vi "OperateOnDigitalOutput.vi"(2 "error in (no error)":errorcluster, 3 "Image Settings":T1={"Start Position (µm)"={"x"=0.0, "y"=0.0, "z"=0.0}, "End Position (µm)"={"x"=10.0, "y"=10.0, "z"=0.0}, "Image Resolution (nm/pixel)"={"x"=50.0, "y"=50.0, "z"=100.0}, "Image Size (µm)"={"x"=10.0, "y"=10.0, "z"=0.0}, "Image Size (pixel)"={"x"=50, "y"=50, "z"=0}, "Time Resolution\n(ms/pixel)"=7.0, "1st Axis"=0, "2nd Axis"=1, "Retrace"=FALSE, "Estimated Time"=""} {"2nd Axis" items=["x", "y", "z"]; "1st Axis" items=["x", "y", "z"]; "Time Resolution\n(ms/pixel)" format="%.2f"; "Image Resolution (nm/pixel)"."z" format="%.2f"; "Image Resolution (nm/pixel)"."y" format="%.2f"; "Image Resolution (nm/pixel)"."x" format="%.2f"; "Image Size (µm)"."z" format="%.2f"; "Image Size (µm)"."y" format="%.2f"; "Image Size (µm)"."x" format="%.2f"; "End Position (µm)"."z" format="%.2f"; "End Position (µm)"."y" format="%.2f"; "End Position (µm)"."x" format="%.2f"; "Start Position (µm)"."z" format="%.2f"; "Start Position (µm)"."y" format="%.2f"; "Start Position (µm)"."x" format="%.2f"}, 4 "operation":enum16{"start", "state", "abort"}(ring)) -> (0 "error out":errorcluster)   [LabVIEW 2009]
uses:
  ImageSettings.ctt
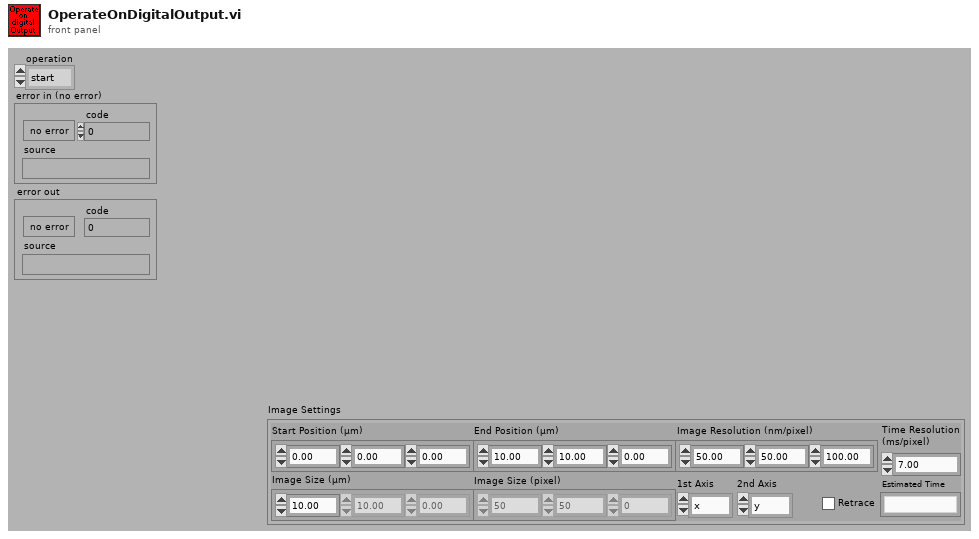
[diagram p1: front panel]
types:
  T1 = typedef "ImageSettings.ctt" = cluster{"Start Position (µm)":cluster{"x":dbl, "y":dbl, "z":dbl}, "End Position (µm)":cluster{"x":dbl, "y":dbl, "z":dbl}, "Image Resolution (nm/pixel)":cluster{"x":dbl, "y":dbl, "z":dbl}, "Image Size (µm)":cluster{"x":dbl, "y":dbl, "z":dbl}, "Image Size (pixel)":cluster{"x":u32, "y":u32, "z":u32}, "Time Resolution\n(ms/pixel)":dbl, "1st Axis":u16, "2nd Axis":u16, "Retrace":bool, "Estimated Time":string}
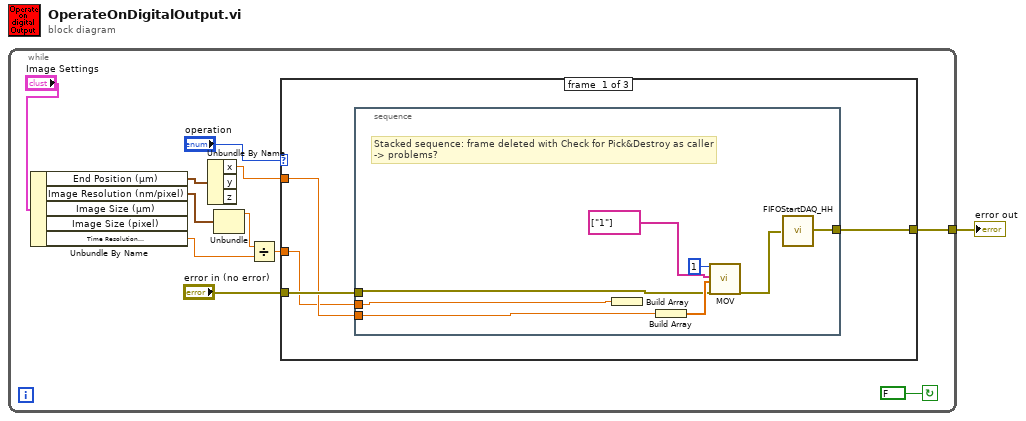
[diagram p0: block diagram]
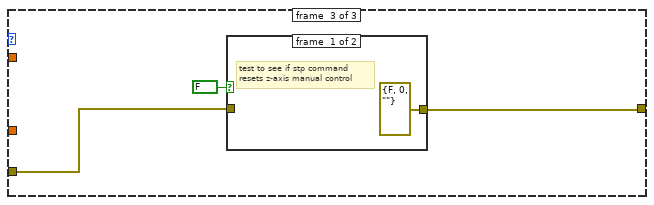
[diagram p3: hidden frame]
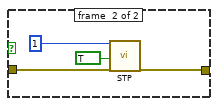
[diagram p4: hidden frame]
diagram:
  n1 = while {
    tunnel: [w9] -> w1
    stop <- FALSE continue-if-true
    n2 = Unbundle By Name("Image Settings") -> ("End Position (µm)"=w7:cluster{"x":dbl, "y":dbl, "z":dbl}, "Image Resolution (nm/pixel)"=w6:cluster{"x":dbl, "y":dbl, "z":dbl}, "Time Resolution\n(ms/pixel)"=w3:dbl)  [unwired: 2 out]
    n3 = Unbundle By Name(w7) -> ("x"=w5:dbl)  [unwired: 2 out]
    n4 = Unbundle(w6) -> ("x"=w4:dbl)  [unwired: 2 out]
    n5 = Divide(x=w4, y=w3) -> (x/y=w2:dbl)
    n6 = case shown="\"abort\"" "operation" {
      tunnel: "error in (no error)" -> [w15 w25 w28]
      tunnel: [w16 w25 w27] -> w9
      tunnel: w5 -> [w14 _ _]
      tunnel: w2 -> [w13 _ _]
      frame #0 {
        n7 = stacked-sequence {
          tunnel: [w24] -> w16
          tunnel: w15 -> [w20]
          tunnel: w14 -> [w23]
          tunnel: w13 -> [w21]
          frame #0 {
            # "Stacked sequence: frame deleted with Check for Pick&Destroy as caller\n-> problems?"
            n8 = Build Array(w21) -> ()  [unwired: 1 out]
            n9 = Build Array(w23) -> (w22:dbl[])
            n10 = call "MOV.vi"("System no."=1, "Axes to move"=string[] ["1"], "Position values"=w22, "error in"=w20) -> ("error out"=w17:errorcluster)  [unwired: 15 in]
            n11 = call "FIFOStartDAQ_HH.vi"("error in (no error)"=w17) -> ("error out"=w24:errorcluster)
          }
        }
      }
      frame #1 {
      }
      frame #2 {
        n12 = case shown="False" FALSE {
          tunnel: w28 -> [_ w33]
          tunnel: [errorcluster {"status"=FALSE, "code"=0, "source"=""} ("error out") w30] -> w27
          frame #0 {
            # "test to see if stp command\nresets z-axis manual control"
          }
          frame #1 {
            n13 = call "STP.vi"("System no."=1, "All axes?"=TRUE, "error in"=w33) -> ("error out"=w30:errorcluster)  [unwired: 16 in]
          }
        }
      }
    }
  }
  "error out" <- w1
